vi "Write Alarms.lvclass.vi"(8 "error in (no error)":errorcluster, 10 "Alarms.lvclass":refnum<class "HK Alarms.lvclass">, 11 "HK Item in":refnum<class "HK Item.lvclass">) -> (0 "error out":errorcluster, 3 "HK Item out":refnum<class "HK Item.lvclass">)   [LabVIEW 2024, in "HK Item.lvclass"]
uses:
  HK Item.lvclass
  HK Alarms/HK Alarms.lvclass
  HK Item.lvclass/HK Item.ctl
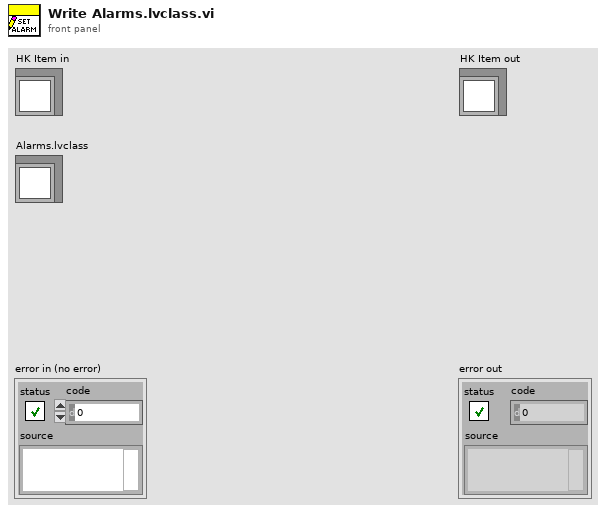
[diagram p1: front panel]
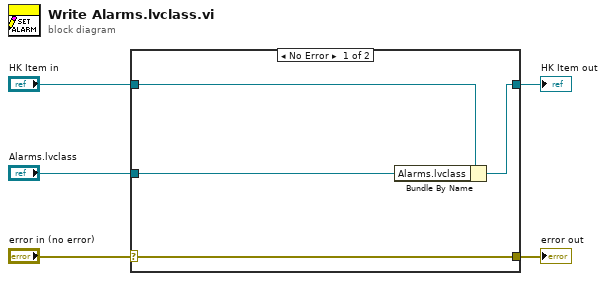
[diagram p0: block diagram]
diagram:
  n1 = case shown="No Error" "error in (no error)" {
    selector: "error in (no error)" -> [w9 w10]
    tunnel: [w9 w10] -> w4
    tunnel: [w7 w11] -> w2
    tunnel: "HK Item in" -> [w8 w11]
    tunnel: "Alarms.lvclass" -> [w6 _]
    frame No Error {
      n2 = Bundle By Name(cluster=w8, "Alarms.lvclass"=w6) -> (w7:refnum<class "HK Item.lvclass">)
    }
    frame Error {
    }
  }
  "error out" <- w4
  "HK Item out" <- w2
